vi "PostFinalTest.vi"(0 "File Path":path[](array[path]), 11 "error in (no error)":errorcluster, 12 "Enable(t)":bool=TRUE) -> (1 "ID":string[](array[string]), 2 "p/f(t = pass)":bool, 3 "name":string[](array[string]), 4 "error?(t)":bool, 6 "Output String":string="REV-C_TETRA_TX-ATTEN database id: 5448\r\nMoved REV-C_TETRA_TX-ATTEN_SN_WAM-000104_2232_060823-120226.csv to Synology Drive\r\nSUCCESS\r\nMoved WAM-C_BOUNCE_SN_WAM-000104_2232_060823-120316_Iq.csv to Synology Drive\r\nWAM-C_BOUNCE database id: 1156\r\nMoved WAM-C_BOUNCE_SN_WAM-000104_2232_060823-120316.csv to Synology Drive\r\nSUCCESS\r\nREV-C_TETRA_TX-PROD-250M database id: 5449\r\nMoved REV-C_TETRA_TX-PROD-250M_SN_WAM-000104_2232_060823-120409.csv to Synology Drive\r\nSUCCESS\r\nCould not move REV-C_TETRA_RX-PROD-250M_SN_WAM-000104_2232_060823-121412_RxCaptureFiles.zip to Synology Drive due to the following error:\r\n[Errno 2] No such file or directory: 'C:\\\\RageATE Results\\\\REV-C_TETRA_RX-PROD-250M\\\\6_8_2023\\\\REV-C_TETRA_RX-PROD-250M_SN_WAM-000104_2232_060823-121412_RxCaptureFiles.zip'\r\nREV-C_TETRA_RX-PROD-250M database id: 5450\r\nMoved REV-C_TETRA_RX-PROD-250M_SN_WAM-000104_2232_060823-121412.csv to Synology Drive\r\nSUCCESS", 15 "error out":errorcluster)   [LabVIEW 2018]
uses:
  Initialize References/Sequence Globals.vi
  <vilib>/regexp/Match Regular Expression.xnode
panel:
  out "file or folder exists?":bool
  out "bounceid":string
  out "Numeric":i32
  out "Numeric 2":i32
  out "attenid":string
  out "txid":string
  out "rxid":string
  out "TX?(t)":bool
  out "Location":string
  out "Message":string
  out "P/F":string
  out "standard error":string
  # "C:\\RageATE Results\\REV-C_TETRA_RX-PROD\\9_6_2022\\REV-C_TETRA_RX-PROD_SN_WAM-000133_2236_090622-175459.csv"
  # "C:\\RageATE Results\\REV-C_TETRA_TX-PROD\\9_6_2022\\REV-C_TETRA_TX-PROD_SN_WAM-000133_2236_090622-173522.csv"
  # "C:\\RageATE Results\\REV-C_TETRA_TX-PROD-250M\\6_7_2023\\REV-C_TETRA_TX-PROD-250M_SN_WAM-000104_ 2232_060723-232333.csv"
  # "C:\\RageATE Results\\REV-C_TETRA_TX-ATTEN\\6_7_2023\\REV-C_TETRA_TX-ATTEN_SN_WAM-000104_ 2232_060723-232242.csv"
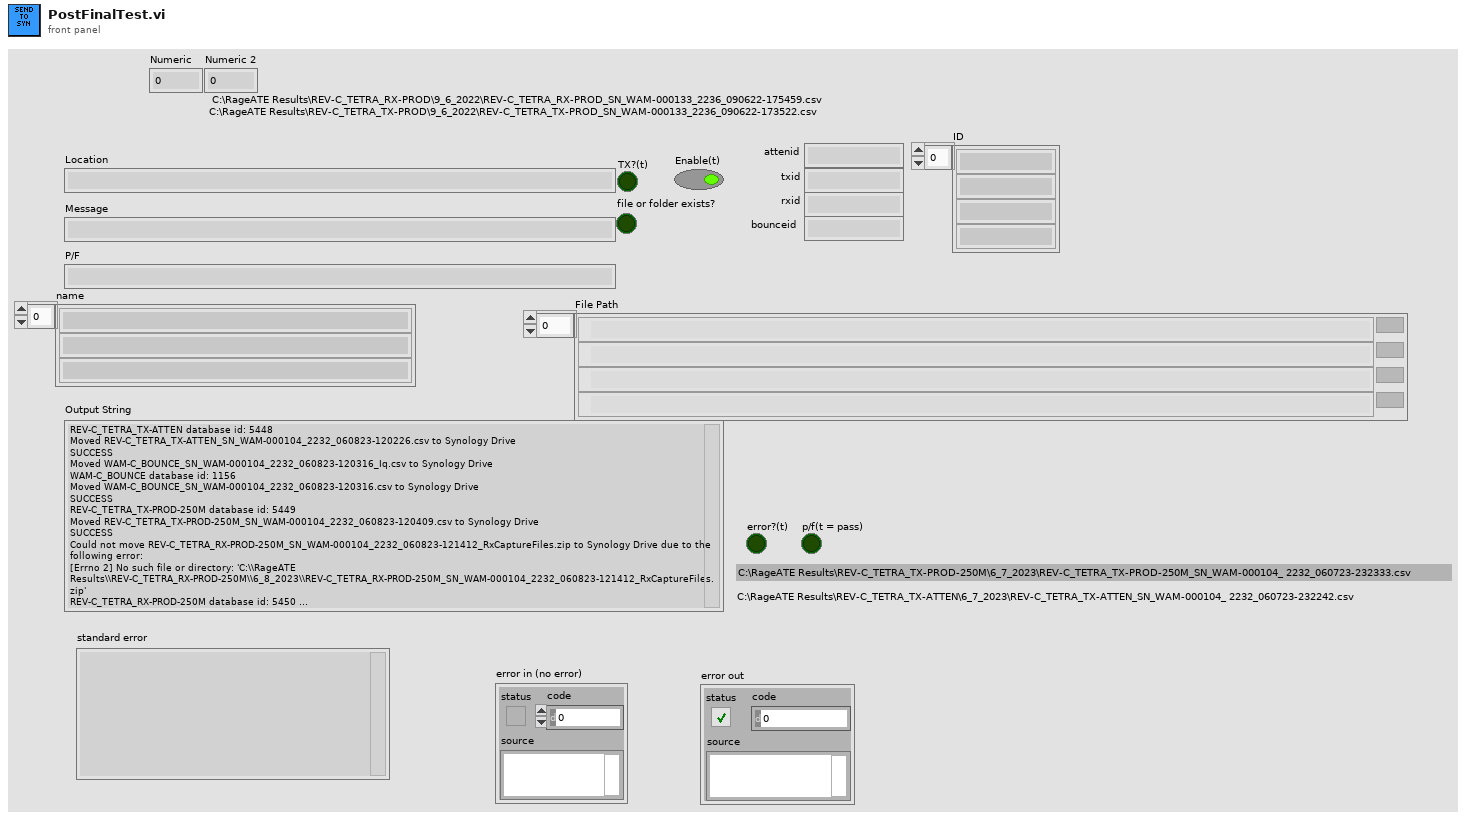
[diagram p1: front panel]
types:
  T1 = enum16{"Left Button", "Center Button", "Right Button", "Window Close"}
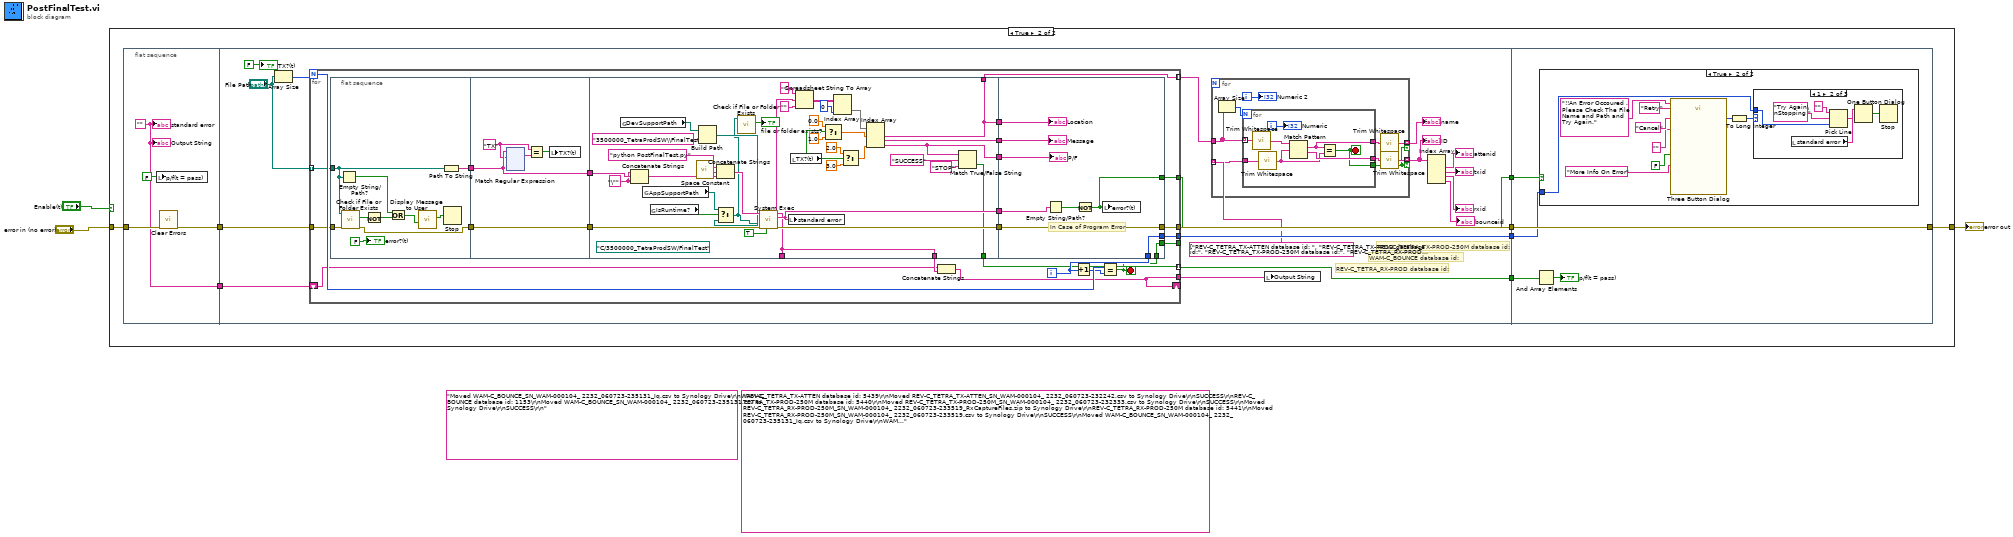
[diagram p0: block diagram]
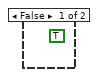
[diagram p3: hidden frame]
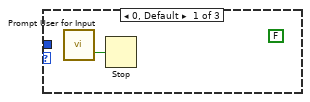
[diagram p4: hidden frame]
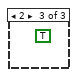
[diagram p5: hidden frame]
diagram:
  (unwired) "REV-C_TETRA_TX-ATTEN database id: 5439\r\nMoved REV-C_TETRA_TX-ATTEN_SN_WAM-000104_ 2232_060723-232242.csv to Synology Drive\r\nSUCCESS\r\nREV-C_TETRA_TX-PROD-250M database id: 5440\r\nMoved REV-C_TETRA_TX-PROD-250M_SN_WAM-000104_ 2232_060723-232333.csv to Synology Drive\r\nSUCCESS\r\nMoved REV-C_TETRA_RX-PROD-250M_SN_WAM-000104_ 2232_060723-233519_RxCaptureFiles.zip to Synology Drive\r\nREV-C_TETRA_RX-PROD-250M database id: 5441\r\nMoved REV-C_TETRA_RX-PROD-250M_SN_WAM-000104_ 2232_060723-233519.csv to Synology Drive\r\nSUCCESS\r\nMoved WAM-C_BOUNCE_SN_WAM-000104_ 2232_060723-235131_Iq.csv to Synology Drive\r\nWAM-C_BOUNCE database id: 1153\r\nMoved WAM-C_BOUNCE_SN_WAM-000104_ 2232_060723-235131.csv to Synology Drive\r\nSUCCESS\r\n" ("standard output")
  (unwired) "Moved WAM-C_BOUNCE_SN_WAM-000104_ 2232_060723-235131_Iq.csv to Synology Drive\r\nWAM-C_BOUNCE database id: 1153\r\nMoved WAM-C_BOUNCE_SN_WAM-000104_ 2232_060723-235131.csv to Synology Drive\r\nSUCCESS\r\n" ("standard output")
  n1 = case shown="True" "Enable(t)" {
    tunnel: [w4 w8] -> w3
    tunnel: "error in (no error)" -> [w4 w7]
    frame False {
    }
    frame True {
      n2 = flat-sequence {
        tunnel: w7 -> [w16]
        tunnel: [w14] -> w6
        tunnel: [w15] -> w5
        tunnel: [w34] -> w12
        tunnel: [w31] -> w11
        tunnel: [w29] -> w10
        tunnel: [w28] -> w9
        tunnel: w6 -> [w27]
        tunnel: w5 -> [w25]
        tunnel: [w254] -> w8
        tunnel: w12 -> [w254]
        tunnel: w11 -> [w253]
        tunnel: w10 -> [w251]
        tunnel: w9 -> [w250]
        frame #0 {
          w15 = ""
          n3 = local write "p/f(t = pass)"(FALSE ("p/f(t = pass)")) -> ()
          n4 = call <vilib>:"Clear Errors.vi"("error in (no error)"=w16) -> ("error out"=w14:errorcluster)  [unwired: 5 in, 1 out]
          "Output String" <- w15
          "standard error" <- w15
        }
        frame #1 {
          # "REV-C_TETRA_RX-PROD database id:"
          # "REV-C_TETRA_TX-PROD-250M database id:"
          # "WAM-C_BOUNCE database id:"
          n5 = Array Size(array="File Path") -> (size(s)=w32:i32)
          n6 = for {
            N: w32 -> [w74]
            tunnel: [w70] -> w34
            tunnel: "File Path" -> [w69] mode=indexing
            tunnel: [w68] -> w31 mode=indexing
            tunnel: [w60] -> w29
            tunnel: [w59] -> _
            tunnel: [w58] -> w28
            tunnel: w27 -> [w56]
            shift-right: [w55] -> _
            shift-left: w25 -> [w53]
            tunnel: [w55] -> w26
            tunnel: [w52] -> w19 mode=indexing
            i -> [w72]
            stop <- w57 stop-if-true
            n7 = flat-sequence {
              tunnel: [w79] -> w64
              tunnel: [w76] -> w62
              tunnel: w69 -> [w78]
              tunnel: w56 -> [w77]
              tunnel: w64 -> [w89]
              tunnel: [w89] -> w63
              tunnel: w62 -> [w90]
              tunnel: [w90] -> w61
              tunnel: w63 -> [w237]
              tunnel: [w236] -> w75
              tunnel: w61 -> [w234]
              tunnel: [w233] -> w71
              tunnel: [w224] -> w68
              tunnel: [w223] -> w67
              tunnel: [w222] -> w66
              tunnel: [w216] -> w65
              tunnel: [w217] -> _
              tunnel: [w217] -> w54
              tunnel: [w216] -> w52
              tunnel: w75 -> [w248]
              tunnel: w57 -> [w242]
              tunnel: w72 -> [w241]
              tunnel: [w247] -> w70
              tunnel: w71 -> [w247]
              tunnel: w67 -> [w246]
              tunnel: w66 -> [w245]
              tunnel: w65 -> [w244]
              tunnel: [w243] -> w60
              tunnel: [w242] -> w59
              tunnel: [w241] -> w58
              frame #0 {
                n8 = Empty String/Path?(string/path=w78) -> (empty?=w81:bool)
                n9 = call <vilib>:"Check if File or Folder Exists.vi"("error in (no error)"=w77, "path"=w78) -> ("error out"=w76:errorcluster, "file or folder exists?"=w80:bool)  [unwired: 7 in, 1 out]
                n10 = Not(x=w80) -> (.not. x?=w82:bool)
                n11 = Or(x=w81, y=w82) -> (x .or. y?=w83:bool)
                n12 = call "Display Message to User"("Enable"=w83) -> ("OK"=w84:bool)  [unwired: 9 in, 1 out]
                n13 = Path To String(path=w78) -> (string=w79:string)
                n14 = Stop(stop? (T)=w84) -> ()
                "error?(t)" <- FALSE ("error?(t)")
              }
              frame #1 {
                w88 = "TX" ("regular expression")
                n15 = xnode "Match Regular Expression"("input string"=w89, "regular expression"=w88) -> ("whole match"=w87:string)  [unwired: 4 in, 4 out]
                n16 = Equal?(x=w88, y=w87) -> (x = y?=w86:bool)
                n17 = local write "TX?(t)"(w86) -> ()
              }
              frame #2 {
                (unwired) path "C:/3500000_TetraProdSW/FinalTest" ("py_path")
                w227 = "\"" ("string")
                n18 = global read "Sequence Globals.vi" "DevSupportPath"() -> (w209:path)
                n19 = Concatenate Strings(w227, w237, w227) -> (w228:string)
                n20 = global read "Sequence Globals.vi" "AppSupportPath"() -> (w210:path)
                n21 = global read "Sequence Globals.vi" "IsRuntime?"() -> (w211:bool)
                n22 = call <vilib>:"Space Constant.vi"() -> ("String"=w238:string)
                n23 = Build Path(base path=w209, name or relative path="3500000_TetraProdSW\\FinalTest") -> (appended path=w208:path)
                n24 = Concatenate Strings("python PostFinalTest.py" ("command line"), w238, w228) -> (w239:string)
                n25 = Select(t=w210, s=w211, f=w208) -> (s? t:f=w206:path)
                n26 = call <vilib>:"Check if File or Folder Exists.vi"("path"=w206) -> ("file or folder exists?"=→"file or folder exists?":bool)  [unwired: 8 in, 2 out]
                n27 = call <vilib>:"System Exec.vi"("run minimized? (F)"=TRUE, "error in (no error)"=w234, "working directory"=w206, "command line"=w239) -> ("error out"=w233:errorcluster, "standard error"=w236:string, "standard output"=w217:string)  [unwired: 4 in, 1 out]
                n28 = local write "standard error"(w236) -> ()
                n29 = local read "TX?(t)"() -> (w212:bool)
                n30 = Spreadsheet String To Array(format string="", spreadsheet string=w217, array type (2D Dbl)="") -> (array=w230:string[][])  [unwired: 1 in]
                n31 = Select(t=0.0, s=w212, f=1.0) -> (s? t:f=w213:dbl)
                n32 = Index Array(array=w230, index (col)=0 ("disabled index (col)")) -> (element=w229:string[])  [unwired: 1 in]
                n33 = Select(t=2.0, s=w212, f=3.0) -> (s? t:f=w220:dbl)
                n34 = Index Array(array=w229, index #1=w213, index #3=w220) -> (element #1=w216:string, element #2=w223:string, element #3=w222:string)  [unwired: 1 in]
                n35 = Match True/False String(2:"STOP" ("false string"), 3:"SUCCESS" ("true string"), 4:w222) -> (0:w224:bool)  [unwired: 1 out]
              }
              frame #3 {
                # "In Case of Program Error"
                n36 = Empty String/Path?(string/path=w248) -> (empty?=w249:bool)
                n37 = Not(x=w249) -> (.not. x?=w243:bool)
                n38 = local write "error?(t)"(w243) -> ()
                "Message" <- w246
                "P/F" <- w245
                "Location" <- w244
              }
            }
            n39 = Concatenate Strings(w53, w54) -> (w55:string)
            n40 = Increment(x=w72) -> (x+1=w73:i32)
            n41 = Equal?(x=w74, y=w73) -> (x = y?=w57:bool)
          }
          n42 = for {
            tunnel: [w39] -> w21 mode=indexing if=w35
            tunnel: [w40] -> w20 mode=indexing if=w35
            tunnel: string[] ["REV-C_TETRA_TX-ATTEN database id: ", "REV-C_TETRA_TX-PROD database id:", "REV-C_TETRA_TX-PROD-250M database id:", "REV-C_TETRA_RX-PROD database id:", "REV-C_TETRA_RX-PROD-250M database id:", "WAM-C_BOUNCE database id:"] ("dbids") -> [w41] mode=indexing
            tunnel: w19 -> [w36]
            i -> [w38]
            n43 = Array Size(array=w36) -> (size(s)=w37:i32)
            n44 = for {
              N: w37 -> [_]
              tunnel: w36 -> [w51] mode=indexing
              tunnel: w41 -> [w50]
              tunnel: [w49] -> w43
              tunnel: [w48] -> w42
              tunnel: [w44] -> w35
              i -> [w45]
              stop <- w44 stop-if-true
              n45 = call <vilib>:"Trim Whitespace.vi"("string"=w51) -> ("trimmed string"=w47:string)  [unwired: 1 in]
              n46 = call <vilib>:"Trim Whitespace.vi"("string"=w50) -> ("trimmed string"=w46:string)  [unwired: 1 in]
              n47 = Match Pattern(string=w47, regular expression=w46) -> (match substring=w48:string, after substring=w49:string)  [unwired: 1 in, 2 out]
              n48 = Equal?(x=w48, y=w46) -> (x = y?=w44:bool)
              "Numeric" <- w45
            }
            n49 = call <vilib>:"Trim Whitespace.vi"("string"=w42) -> ("trimmed string"=w40:string)  [unwired: 1 in]
            n50 = call <vilib>:"Trim Whitespace.vi"("string"=w43) -> ("trimmed string"=w39:string)  [unwired: 1 in]
            "Numeric 2" <- w38
          }
          "ID" <- w21
          "name" <- w20
          n51 = local write "Output String"(w26) -> ()
          n52 = Index Array(array=w21) -> (element #1=→"attenid":string, element #2=→"txid":string, element #3=→"rxid":string, element #4=→"bounceid":string)  [unwired: 4 in]
          "TX?(t)" <- FALSE ("TX?(t)")
        }
        frame #2 {
          n53 = And Array Elements(Boolean array=w253) -> (logical AND=→"p/f(t = pass)":bool)
          n54 = case shown="True" w251 {
            tunnel: w250 -> [_ w255]
            frame False {
              (unwired) TRUE
            }
            frame True {
              n55 = call <vilib>:"Three Button Dialog.vi"("Allow user to close window? (TRUE)"=FALSE, "Window Title (\"\")"="" ("Window Title (\"\")"), "Right Button Text (\"Cancel\")"="Cancel" ("Right Button Text (\"Cancel\")"), "Center Button Text (\"No\")"="More Info On Error" ("Center Button Text (\"No\")"), "Left Button Text (\"Yes\")"="Retry" ("Left Button Text (\"Yes\")"), "message"="!!An Error Occoured . Please Check The File Name and Path and Try Again." ("Message")) -> ("Which Button?"=w257:T1)  [unwired: 5 in]
              n56 = To Long Integer(number=w257) -> (32bit integer=w256:i32)
              n57 = case shown="1" w256 {
                tunnel: w255 -> [_ w266 _]
                frame 0, Default {
                  (unwired) FALSE
                  n58 = call "Prompt User for Input"() -> ("OK"=w264:bool)  [unwired: 18 in, 1 out]
                  n59 = Stop(stop? (T)=w264) -> ()
                }
                frame 1 {
                  n60 = local read "standard error"() -> (w270:string)
                  n61 = Pick Line(string ("")="", multi-line string="Try Again\nStopping " ("button name (\"OK\")"), line index=w266) -> (output string=w269:string)
                  n62 = One Button Dialog(message=w270, button name ("OK")=w269) -> (true=w265:bool)
                  n63 = Stop(stop? (T)=w265) -> ()
                }
                frame 2 {
                  (unwired) TRUE
                }
              }
            }
          }
        }
      }
    }
  }
  "error out" <- w3
